vi "LitePoint_PortConfiguration.vi"() -> ()   [LabVIEW 2020, in "LitePoints.lvlib"]
uses:
  LitePoints.lvlib
panel:
  out "read buffer":string
  out "error out":errorcluster
  out "VISA resource name out":refnum<visa-resource-name>
  in  "VISA resource name":refnum<visa-resource-name>
  in  "error in (no error)":errorcluster
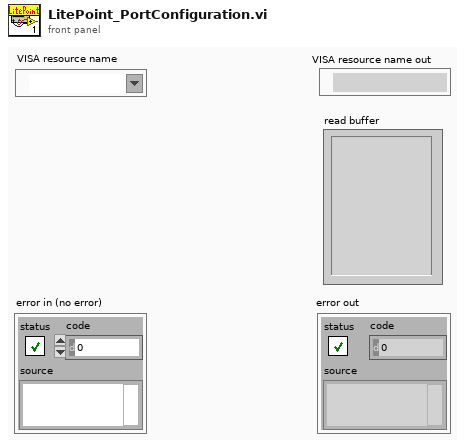
[diagram p1: front panel]
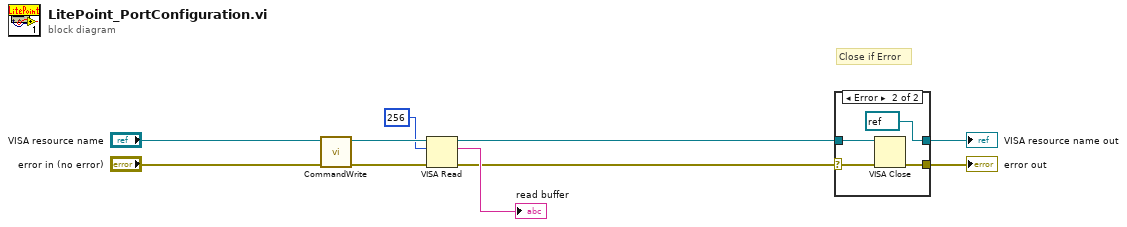
[diagram p0: block diagram]
diagram:
  # "Close if Error"
  n1 = call "CommandWrite.vi"("error in (no error)"="error in (no error)", "VISA resource name"="VISA resource name") -> ("error out"=w7:errorcluster, "VISA resource name out"=w8:refnum<visa-resource-name>)  [unwired: 8 in]
  n2 = VISA Read(VISA resource name=w8, byte count=u32 256, error in (no error)=w7) -> (VISA resource name out=w4:refnum<visa-resource-name>, read buffer=→"read buffer":string, error out=w3:errorcluster)  [unwired: 1 out]
  n3 = case shown="Error" w3 {
    selector: w3 -> [w11 w14]
    tunnel: w4 -> [w12 w15]
    tunnel: [w12 refnum<visa-resource-name> refnum ("VISA resource name out")] -> w10
    tunnel: [w11 w13] -> w9
    frame No Error {
    }
    frame Error {
      n4 = VISA Close(VISA resource name=w15, error in (no error)=w14) -> (error out=w13:errorcluster)
    }
  }
  "VISA resource name out" <- w10
  "error out" <- w9
